vi "speedOfLoop.vi"() -> ()   [LabVIEW 2021]
panel:
  in  "Freq":dbl(knob) scale=1.0..100.0
  out "Waveform Chart":dbl(graph)
  in  "Stop":bool
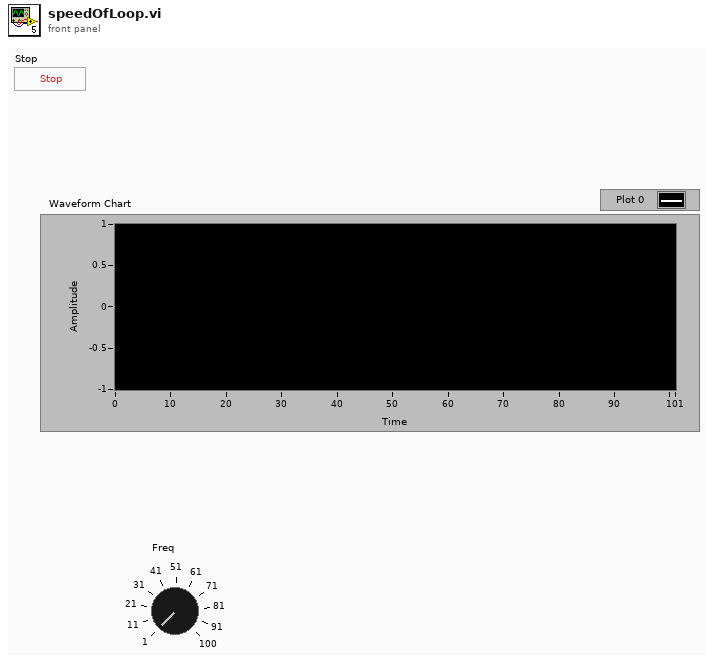
[diagram p1: front panel]
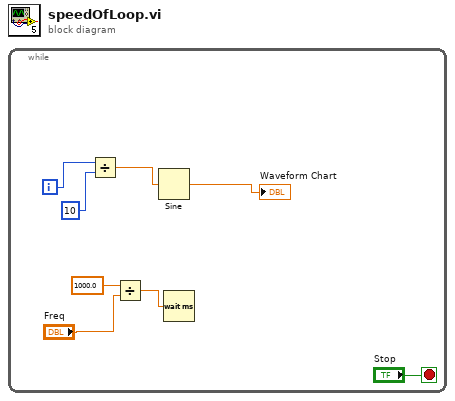
[diagram p0: block diagram]
diagram:
  n1 = while {
    i -> [w7]
    stop <- "Stop" stop-if-true
    n2 = Divide(x=w7, y=10) -> (x/y=w5:dbl)
    n3 = Divide(x=1000.0, y="Freq") -> (x/y=w1:dbl)
    n4 = Sine(x=w5) -> (sin(x)=→"Waveform Chart":dbl)
    n5 = Wait (ms)(milliseconds to wait=w1) -> ()  [unwired: 1 out]
  }
